vi "cRIO IV PID test.vi"(1 "AI Chan":i32, 2 "AO Channel":string(combo)="AO0", 7 "Voltage target V":dbl=1e-05, 12 "delay s":dbl=0.05 format="%.3f", 13 "error":dbl) -> (4 "I Output uA":dbl, 15 "error out":errorcluster)   [LabVIEW 2021]
uses:
  <vilib>/addons/control/pid/NI_PID_pid.lvlib
  <vilib>/addons/control/pid/pid.llb/PID (DBL).vi
panel:
  in  "Init Current uA":dbl=3.0 format="%#_13g"
  out "Voltage":cluster{"t0":dbl, "dt":dbl, dbl[][]}(graph)={"t0"=0.0, "dt"=0.23150301830064327, [[-6.2742919921875e-06, 7.0286865234375e-06, 7.5959472656250004e-06, 7.587646484375001e-06, 6.8331298828125e-06, 8.3389892578125e-06, 7.4207763671875e-06, 8.2294921875e-06, 6.97802734375e-06, 8.307373046875e-06, 7.221801757812501e-06, 7.378784179687501e-06, 8.218017578125e-06, 7.3470458984375005e-06, 8.3358154296875e-06, 7.828613281250001e-06, 9.2227783203125e-06, 9.056640625e-06, 8.68896484375e-06, 7.5644531249999994e-06, 8.111450195312501e-06, 9.3924560546875e-06, 9.149658203125e-06, 8.9468994140625e-06, 8.8182373046875e-06, 9.553344726562501e-06, 7.7969970703125e-06, 7.2528076171875e-06, 8.03564453125e-06, 9.9212646484375e-06, 9.2659912109375e-06, 8.3221435546875e-06, 8.722412109375e-06, 7.700927734375e-06, 9.4189453125e-06, 7.7850341796875e-06, 7.683349609375e-06, 1.14346923828125e-05, 1.01173095703125e-05, 9.098388671875e-06, 8.264038085937501e-06, 1.0583740234375e-05, 9.461791992187501e-06, 9.5201416015625e-06, 7.613403320312501e-06, 8.979125976562501e-06, 1.012158203125e-05, 8.5411376953125e-06, 8.268920898437501e-06, 8.615234375e-06, 8.764404296875e-06, 9.4747314453125e-06, 8.604370117187501e-06, 7.9896240234375e-06, 8.267822265625e-06, 8.7490234375e-06, 8.952026367187501e-06, 9.116943359375e-06, 1.1099365234375e-05, 9.396484375e-06, 9.9132080078125e-06, 1.0455322265625e-05, 1.02037353515625e-05, 9.993408203125e-06, 9.0792236328125e-06, 1.05933837890625e-05, 8.10009765625e-06, 1.131103515625e-05, 9.5404052734375e-06, 8.3836669921875e-06, 9.6424560546875e-06, 8.5926513671875e-06, 1.0763916015625e-05, 1.0721557617187499e-05, 9.448974609375e-06, 1.0819946289062501e-05, 8.394897460937502e-06, 1.03946533203125e-05, 9.9185791015625e-06, 9.932739257812501e-06, 9.6884765625e-06, 9.885986328125e-06, 9.747802734375e-06, 9.4522705078125e-06, 9.875122070312501e-06, 1.064501953125e-05, 1.02010498046875e-05, 9.4254150390625e-06, 1.05379638671875e-05, 1.062939453125e-05, 1.03377685546875e-05, 7.7686767578125e-06, 1.03857421875e-05, 8.9049072265625e-06, 1.01602783203125e-05, 1.0444458007812501e-05, 9.0526123046875e-06, 9.9517822265625e-06, 9.619873046875e-06, 9.9910888671875e-06, 9.627685546875001e-06, 1.16241455078125e-05, 1.01810302734375e-05, 8.827880859375e-06, 9.647827148437501e-06, 8.648193359375e-06, 9.631225585937501e-06, 1.1260375976562501e-05, 9.3602294921875e-06, 1.1323364257812501e-05, 1.00931396484375e-05, 9.7305908203125e-06, 1.0537109375000001e-05, 9.133178710937501e-06, 1.06405029296875e-05, 9.4534912109375e-06, 9.677490234375e-06, 1.0020385742187501e-05, 1.0294677734375e-05, 9.501953125e-06, 1.1838745117187502e-05, 1.01229248046875e-05, 1.0786132812500001e-05, 9.9029541015625e-06, 9.881469726562501e-06, 1.03533935546875e-05, 1.02386474609375e-05, 9.5933837890625e-06, 1.1360473632812501e-05, 8.740966796875e-06, 9.8046875e-06, 9.3798828125e-06, 9.642578124999999e-06, 1.087841796875e-05, 9.199951171875e-06, 1.0077880859375e-05, 1.04891357421875e-05, 9.737548828125001e-06, 9.2452392578125e-06, 9.141235351562501e-06, 1.0398071289062499e-05, 8.7894287109375e-06, 9.27197265625e-06, 9.757934570312501e-06, 1.03651123046875e-05, 9.6182861328125e-06, 9.383544921875001e-06, 1.01751708984375e-05, 1.06143798828125e-05, 8.880126953125e-06, 9.0814208984375e-06, 9.64013671875e-06, 9.750732421875e-06, 1.0253662109375e-05, 1.0913940429687502e-05, 9.9195556640625e-06, 1.0969360351562501e-05, 1.1051513671875e-05, 1.05164794921875e-05, 1.0513549804687501e-05, 1.0940307617187501e-05, 9.00634765625e-06, 9.565185546875001e-06, 1.08887939453125e-05, 9.060424804687501e-06, 1.09468994140625e-05, 9.7672119140625e-06, 9.77978515625e-06, 9.439208984375e-06, 8.5277099609375e-06, 1.17899169921875e-05, 1.0476074218750001e-05, 9.598754882812501e-06, 9.685546875000001e-06, 9.630859375000001e-06, 8.735229492187501e-06, 1.0571533203125e-05, 1.01201171875e-05, 9.3568115234375e-06, 1.1734130859375e-05, 1.00394287109375e-05, 9.65185546875e-06, 1.0709838867187501e-05, 9.6763916015625e-06, 1.07955322265625e-05, 8.813720703125e-06, 1.09769287109375e-05, 9.6085205078125e-06, 1.07159423828125e-05, 9.62841796875e-06, 1.0301025390625e-05, 9.542236328125e-06, 1.00299072265625e-05, 9.475219726562501e-06, 1.0421630859375e-05, 1.03519287109375e-05, 9.370117187500001e-06, 9.962646484375e-06, 9.717651367187501e-06, 1.0513427734375001e-05, 9.867187500000002e-06, 1.02030029296875e-05, 9.1756591796875e-06, 1.0221191406250002e-05, 8.7371826171875e-06, 9.9151611328125e-06, 9.8636474609375e-06, 1.0983642578125e-05, 1.06876220703125e-05, 9.659912109375001e-06, 8.753662109375001e-06, 9.053833007812502e-06, 1.0186401367187501e-05, 1.0432128906250001e-05, 1.0882812500000001e-05, 1.1218994140625e-05, 1.1887451171875001e-05, 1.0174072265625e-05, 9.899658203125e-06, 1.0531494140625e-05, 9.444824218750001e-06, 8.6407470703125e-06, 9.7640380859375e-06, 9.9656982421875e-06, 1.0595336914062502e-05, 9.55712890625e-06, 1.1597534179687501e-05, 9.322753906250001e-06, 1.0935424804687501e-05, 9.472045898437501e-06, 1.0580322265625e-05, 1.0116943359375001e-05, 9.96728515625e-06, 1.1901245117187501e-05, 1.0048583984375e-05, 1.0146484375000002e-05, 1.0034179687500001e-05, 1.044482421875e-05, 9.5802001953125e-06, 1.0305175781250001e-05, 9.824462890625001e-06, 9.204833984375e-06, 9.7882080078125e-06, 8.905517578125e-06, 8.972412109375e-06, 1.04232177734375e-05, 1.0131591796875e-05, 1.0323852539062501e-05, 1.0559326171875e-05, 1.06358642578125e-05, 1.0219482421875e-05, 1.0810424804687502e-05, 9.529907226562502e-06, 1.01871337890625e-05, 9.165283203125001e-06, 9.7891845703125e-06, 1.0254150390625001e-05, 1.0550781250000001e-05, 1.0967407226562501e-05, 9.429077148437499e-06, 9.159179687500002e-06, 9.6815185546875e-06, 1.1452514648437502e-05, 1.0664794921875e-05, 9.7794189453125e-06, 9.3082275390625e-06, 1.2046142578125e-05, 9.310546875e-06, 1.092138671875e-05, 9.867431640625e-06, 9.5145263671875e-06, 1.0375e-05, 1.0604858398437501e-05, 9.5135498046875e-06, 1.0877685546875001e-05, 8.9964599609375e-06, 9.785400390625001e-06, 1.0837646484375002e-05, 9.8760986328125e-06, 9.861572265625001e-06, 1.04326171875e-05, 1.1680419921875001e-05, 9.5611572265625e-06, 8.8084716796875e-06, 1.0350341796875e-05, 1.10693359375e-05, 8.979736328125e-06, 1.01485595703125e-05, 1.1346923828125e-05, 8.6527099609375e-06, 9.1024169921875e-06, 8.1697998046875e-06, 1.1321289062500001e-05, 8.2783203125e-06, 9.943603515625e-06, 8.751220703125e-06, 1.04207763671875e-05, 1.1733642578125002e-05, 1.1821533203125e-05, 1.08138427734375e-05, 1.00948486328125e-05, 9.882446289062502e-06, 9.6370849609375e-06, 8.97802734375e-06, 9.022216796875e-06, 9.816650390625e-06], [1e-05, 1e-05, 1e-05, 1e-05, 1e-05, 1e-05, 1e-05, 1e-05, 1e-05, 1e-05, 1e-05, 1e-05, 1e-05, 1e-05, 1e-05, 1e-05, 1e-05, 1e-05, 1e-05, 1e-05, 1e-05, 1e-05, 1e-05, 1e-05, 1e-05, 1e-05, 1e-05, 1e-05, 1e-05, 1e-05, 1e-05, 1e-05, 1e-05, 1e-05, 1e-05, 1e-05, 1e-05, 1e-05, 1e-05, 1e-05, 1e-05, 1e-05, 1e-05, 1e-05, 1e-05, 1e-05, 1e-05, 1e-05, 1e-05, 1e-05, 1e-05, 1e-05, 1e-05, 1e-05, 1e-05, 1e-05, 1e-05, 1e-05, 1e-05, 1e-05, 1e-05, 1e-05, 1e-05, 1e-05, 1e-05, 1e-05, 1e-05, 1e-05, 1e-05, 1e-05, 1e-05, 1e-05, 1e-05, 1e-05, 1e-05, 1e-05, 1e-05, 1e-05, 1e-05, 1e-05, 1e-05, 1e-05, 1e-05, 1e-05, 1e-05, 1e-05, 1e-05, 1e-05, 1e-05, 1e-05, 1e-05, 1e-05, 1e-05, 1e-05, 1e-05, 1e-05, 1e-05, 1e-05, 1e-05, 1e-05, 1e-05, 1e-05, 1e-05, 1e-05, 1e-05, 1e-05, 1e-05, 1e-05, 1e-05, 1e-05, 1e-05, 1e-05, 1e-05, 1e-05, 1e-05, 1e-05, 1e-05, 1e-05, 1e-05, 1e-05, 1e-05, 1e-05, 1e-05, 1e-05, 1e-05, 1e-05, 1e-05, 1e-05, 1e-05, 1e-05, 1e-05, 1e-05, 1e-05, 1e-05, 1e-05, 1e-05, 1e-05, 1e-05, 1e-05, 1e-05, 1e-05, 1e-05, 1e-05, 1e-05, 1e-05, 1e-05, 1e-05, 1e-05, 1e-05, 1e-05, 1e-05, 1e-05, 1e-05, 1e-05, 1e-05, 1e-05, 1e-05, 1e-05, 1e-05, 1e-05, 1e-05, 1e-05, 1e-05, 1e-05, 1e-05, 1e-05, 1e-05, 1e-05, 1e-05, 1e-05, 1e-05, 1e-05, 1e-05, 1e-05, 1e-05, 1e-05, 1e-05, 1e-05, 1e-05, 1e-05, 1e-05, 1e-05, 1e-05, 1e-05, 1e-05, 1e-05, 1e-05, 1e-05, 1e-05, 1e-05, 1e-05, 1e-05, 1e-05, 1e-05, 1e-05, 1e-05, 1e-05, 1e-05, 1e-05, 1e-05, 1e-05, 1e-05, 1e-05, 1e-05, 1e-05, 1e-05, 1e-05, 1e-05, 1e-05, 1e-05, 1e-05, 1e-05, 1e-05, 1e-05, 1e-05, 1e-05, 1e-05, 1e-05, 1e-05, 1e-05, 1e-05, 1e-05, 1e-05, 1e-05, 1e-05, 1e-05, 1e-05, 1e-05, 1e-05, 1e-05, 1e-05, 1e-05, 1e-05, 1e-05, 1e-05, 1e-05, 1e-05, 1e-05, 1e-05, 1e-05, 1e-05, 1e-05, 1e-05, 1e-05, 1e-05, 1e-05, 1e-05, 1e-05, 1e-05, 1e-05, 1e-05, 1e-05, 1e-05, 1e-05, 1e-05, 1e-05, 1e-05, 1e-05, 1e-05, 1e-05, 1e-05, 1e-05, 1e-05, 1e-05, 1e-05, 1e-05, 1e-05, 1e-05, 1e-05, 1e-05, 1e-05, 1e-05, 1e-05, 1e-05, 1e-05, 1e-05, 1e-05, 1e-05, 1e-05, 1e-05, 1e-05, 1e-05, 1e-05, 1e-05, 1e-05, 1e-05, 1e-05, 1e-05, 1e-05, 1e-05, 1e-05, 1e-05, 1e-05, 1e-05, 1e-05, 1e-05, 1e-05, 1e-05, 1e-05, 1e-05, 1e-05, 1e-05, 1e-05, 1e-05, 1e-05, 1e-05]]}
  out "Current":T1(graph)={"t0"=0.0, "dt"=0.23150301830064327, "Current array"=[3.006509716796875, 3.0076982428290204, 3.008659864605964, 3.00962480673273, 3.0108915555432136, 3.011555960640877, 3.012587650927396, 3.0132958549192814, 3.0145046448855526, 3.015181696606828, 3.0162929768781503, 3.017341464222326, 3.0180542582410417, 3.019115440965791, 3.019781115911303, 3.0206496717457356, 3.020960561587261, 3.021337906520166, 3.021862321782928, 3.0228365417620404, 3.0235919629463752, 3.0238349818062042, 3.024175119817897, 3.024596361359919, 3.025069067762951, 3.0252477312098036, 3.02612893373961, 3.0272278120888694, 3.028013555708861, 3.0280450512977475, 3.028338656267904, 3.029009800319169, 3.029520836971361, 3.030440467401184, 3.0306728908220024, 3.0315588787175365, 3.032485540476193, 3.0319116651322875, 3.031864742901392, 3.032225389035931, 3.0329197754252206, 3.032686280964038, 3.032901565799378, 3.033093510798843, 3.03404815113298, 3.0344565024309724, 3.034407871314046, 3.0349914179418387, 3.0356838513130504, 3.036237759317731, 3.036731999373934, 3.0369421085843813, 3.037500362340937, 3.038304514561335, 3.0389973875138043, 3.0394977800205947, 3.039916971373285, 3.0402701959440295, 3.039830451763102, 3.040071859922092, 3.0401065786332917, 3.0399244516385187, 3.0398429594042793, 3.039845598027892, 3.0402139104867927, 3.039976558885723, 3.04073652174787, 3.0402121096145653, 3.040395949427809, 3.041042484569587, 3.041185504101611, 3.041748445522266, 3.041442881088515, 3.041154260002669, 3.041374672118631, 3.041046695560642, 3.041688738539966, 3.0415308791848856, 3.041563449514887, 3.041590355783536, 3.041714967133234, 3.041760574579968, 3.0418614554670294, 3.0420805492508913, 3.042130502414945, 3.0418724965906057, 3.0417920786503556, 3.0420219146192404, 3.041806731057158, 3.0415549752204347, 3.041419869766867, 3.0423124010466727, 3.0421581061688574, 3.0425961452808954, 3.042532035962653, 3.0423542547647404, 3.0427332118519614, 3.0427525009781196, 3.0429045537794606, 3.042908120255681, 3.0430570480629706, 3.042407391876219, 3.0423349817692773, 3.0428038314356147, 3.0429447025980987, 3.0434854272893648, 3.043632939103291, 3.0431287907540807, 3.043384700993828, 3.042855357322046, 3.042818103483074, 3.042925869176714, 3.042711027446411, 3.0430577579842795, 3.0428015588363957, 3.043020164375286, 3.043149170311513, 3.043141018046948, 3.0430231489830746, 3.0432223697645218, 3.042486873738742, 3.042437705822814, 3.0421232546967416, 3.042162075049723, 3.042209489154369, 3.0420681337259516, 3.0419726767304627, 3.0421353252050207, 3.0415911377347116, 3.0420947529979934, 3.042172879991262, 3.0424209288658304, 3.0425638996229516, 3.0422125344385478, 3.0425325559722887, 3.0425014056366084, 3.042305753343423, 3.0424107358141113, 3.0427126421207817, 3.043056150002415, 3.0428969235126067, 3.043381154060324, 3.04367236704489, 3.043769195271324, 3.043623152403058, 3.04377584000367, 3.044022424096366, 3.0439523578018455, 3.0437066079074775, 3.0441545591888883, 3.044521992907921, 3.0446659403087035, 3.044765649432941, 3.044664186682145, 3.0442986125942055, 3.044330792406079, 3.043943050336085, 3.043522446922355, 3.0433158571683876, 3.0431104392814636, 3.0427343182583098, 3.043131781219943, 3.04330570903636, 3.0429501934898946, 3.0433260256000714, 3.0429472678664418, 3.0430403851272954, 3.0431284730947734, 3.043352791537035, 3.0439417096043764, 3.0432257448567643, 3.0430353172010234, 3.0431958172790794, 3.043321600565789, 3.0434692588577787, 3.043975169115514, 3.043746557894229, 3.043698513073852, 3.0439557905231394, 3.0432621402296256, 3.0432463707817887, 3.043385630633211, 3.0431016971224643, 3.043231142514984, 3.0429129316538583, 3.043387445405126, 3.042996675954886, 3.0431532697813735, 3.0428668948553548, 3.043015529692301, 3.0428951215610427, 3.0430782290559946, 3.043066268194876, 3.0432761823375802, 3.043107532027956, 3.042966762571732, 3.04321871772703, 3.043233661168731, 3.043346602659777, 3.043141233602163, 3.0431943606353595, 3.043113161496139, 3.043442899861717, 3.043354425341327, 3.0438595543446056, 3.043893491952041, 3.0439480350299344, 3.04355458005441, 3.043279533269107, 3.0434155704654953, 3.043914107674133, 3.044292576540325, 3.0442180180686322, 3.0440451685765395, 3.043692045636795, 3.0432044500245703, 3.0424494715758597, 3.042379844673732, 3.0424199833960346, 3.042207387740009, 3.042429460052916, 3.0429731632399806, 3.043067550033112, 3.0430812727658303, 3.0428431400254667, 3.043020290487051, 3.0423812788303457, 3.04265217927591, 3.0422780113601062, 3.0424891950036566, 3.0422570680999272, 3.0422102927533152, 3.042223380687303, 3.041462884622491, 3.041443452995752, 3.0413848612112573, 3.0413711913003674, 3.0411932635732795, 3.0413611854553735, 3.041239117103977, 3.0413093339078303, 3.041627402281677, 3.041712121053922, 3.0421499160081256, 3.0425609531662103, 3.042391668063335, 3.0423390333468023, 3.042209494329879, 3.041985765853014, 3.0417314221325484, 3.041643631139856, 3.0413194631860896, 3.0415075022609463, 3.041432650712987, 3.0417665394044007, 3.0418508675570086, 3.041749209381157, 3.041528898855343, 3.041141937927185, 3.041370309027216, 3.0417066391225194, 3.041834033679897, 3.0412530297910196, 3.0409871137764224, 3.0410753481490214, 3.041352059091163, 3.040533604007225, 3.0408093871940642, 3.040440834441613, 3.040493863714323, 3.0406880551011786, 3.0405380570357616, 3.040296115603407, 3.0404906976076385, 3.0401396253119755, 3.0405410432516584, 3.0406268850288685, 3.04029182836377, 3.0403413908337873, 3.0403967638527045, 3.040223718900601, 3.0395515528384407, 3.039727091844824, 3.040203705082539, 3.040063570279871, 3.039635837809997, 3.0400439451834944, 3.0399845232668437, 3.0394457556355263, 3.039984673551087, 3.0403437086714717, 3.041075790687906, 3.040547277005143, 3.04123595082547, 3.041258511378268, 3.0417580250661387, 3.041589716494774, 3.0408962614224078, 3.0401676500726067, 3.039842114874344, 3.039804177325319, 3.0398512007139695, 3.0399963686375773, 3.040405159618747, 3.0407962748340984, 3.04086961662091]}
  in  "Average":i32=200
  out "Current uA":dbl=3.04086961662091
  in  "Stop":bool
  in  "I Scale factor":dbl=10.0
  in  "V Scale factor":dbl=0.0001
  in  "PID gains":T2={"proportional gain (Kc)"=400.0, "integral time (Ti, min)"=100000.0, "derivative time (Td, min)"=0.0} {"derivative time (Td, min)" format="%.3f"; "integral time (Ti, min)" format="%.3f"; "proportional gain (Kc)" format="%.3f"}
  # "Voltage x factor=actual"
  # "Voltage x factor=uA"
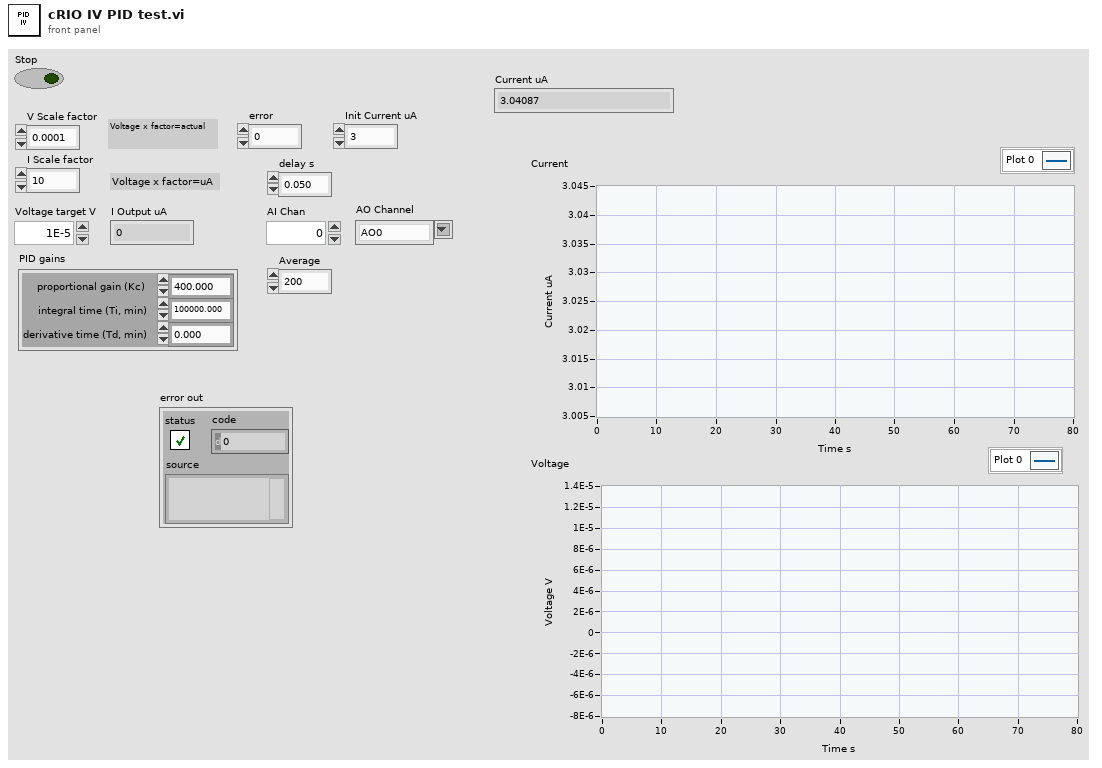
[diagram p1: front panel]
types:
  T1 = cluster{"t0":dbl, "dt":dbl, "Current array":dbl[]}
  T2 = cluster{"proportional gain (Kc)":dbl, "integral time (Ti, min)":dbl, "derivative time (Td, min)":dbl}
  T3 = cluster{"AI0":dbl, "AI1":dbl, "AI2":dbl, "AI3":dbl}
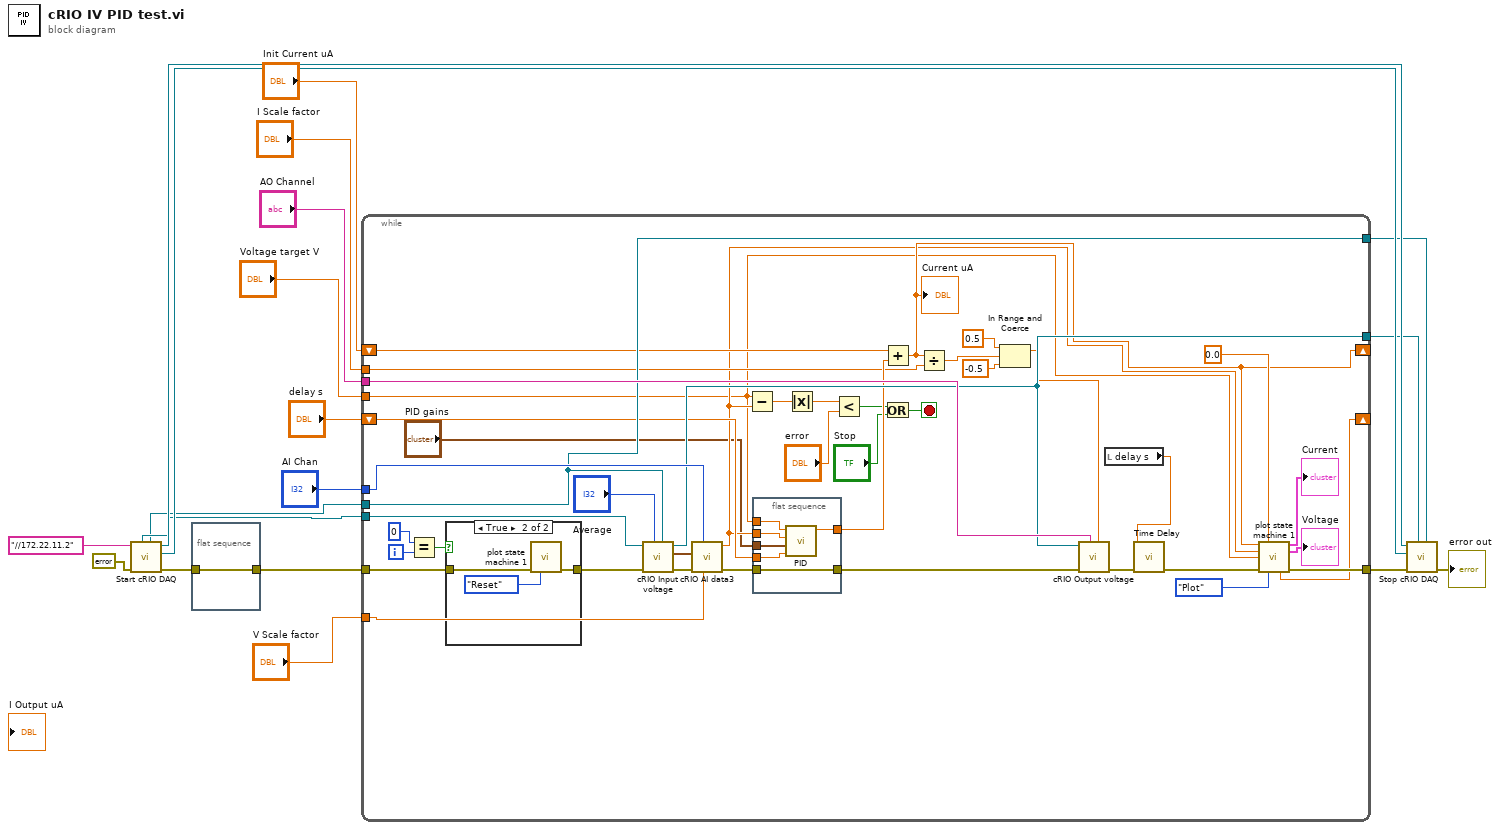
[diagram p0: block diagram]
diagram:
  n1 = call "Start cRIO DAQ.vi"("error in (no error)"=errorcluster {"status"=FALSE, "code"=0, "source"=""}, "cRIO IP"="//172.22.11.2") -> ("error out"=w3:errorcluster, "vi reference"=w9:refnum<vi>, "application reference"=w10:refnum<vi>, "DAQ_AI_Reader endpoint"=w7:refnum<k21>, "DAQ_CMD_Writer endpoint"=w8:refnum<k21>)  [unwired: 5 in]
  n2 = flat-sequence {
    tunnel: [w20] -> w2
    tunnel: w3 -> [w20]
    frame #0 {
    }
  }
  n3 = while {
    tunnel: w2 -> [w33]
    tunnel: [w37] -> w12
    tunnel: "Voltage target V" -> [w26]
    tunnel: w8 -> [w59]
    tunnel: w7 -> [w50]
    tunnel: "V Scale factor" -> [w61]
    tunnel: "AI Chan" -> [w58]
    tunnel: "AO Channel" -> [w57]
    tunnel: "I Scale factor" -> [w48]
    tunnel: [w51] -> w5
    tunnel: [w50] -> w4
    shift-right: [w28] -> _
    shift-left: "Init Current uA" -> [w39]
    shift-right: [w22] -> _
    shift-left: "delay s" -> [w29]
    i -> [w36]
    stop <- w41 stop-if-true
    n4 = Equal?(x=0, y=w36) -> (x = y?=w34:bool)
    n5 = case shown="True" w34 {
      tunnel: w33 -> [w64 w67]
      tunnel: [w64 w66] -> w32
      frame False {
      }
      frame True {
        n6 = call "plot state machine 1.vi"("error in"=w67, "Enum"=enum16{"Reset", "Plot"}."Reset") -> ("error out"=w66:errorcluster)  [unwired: 10 in, 3 out]
      }
    }
    n7 = call "cRIO Input voltage.vi"("DAQ_AI_Reader endpoint"=w50, "Average"="Average", "error in (no error)"=w32, "DAQ_CMD_Writer endpoint"=w59) -> ("error out"=w62:errorcluster, "output cluster"=w63:T3, "DAQ_CMD_Writer endpoint out"=w51:refnum<k21>)  [unwired: 5 in]
    n8 = call "cRIO AI data3.vi"("Scale factor"=w61, "Chan"=w58, "error in (no error)"=w62, "Input cluster"=w63) -> ("error out"=w60:errorcluster, "Output"=w27:dbl)  [unwired: 6 in]
    n9 = Subtract(x=w26, y=w27) -> (x-y=w54:dbl)
    n10 = flat-sequence {
      tunnel: "PID gains" -> [w73]
      tunnel: w29 -> [w72]
      tunnel: w26 -> [w68]
      tunnel: w27 -> [w71]
      tunnel: w60 -> [w70]
      tunnel: [w70] -> w56
      tunnel: [w69] -> w49
      frame #0 {
        n11 = call-poly <vilib>:"PID.vi"("dt (s)"=w72, "PID gains"=w73, "process variable"=w71, "setpoint"=w68) -> ("output"=w69:dbl)  [unwired: 6 in, 1 out]
      }
    }
    n12 = Absolute Value(x=w54) -> (abs(x)=w53:dbl)
    n13 = Less?(x=w53, y="error") -> (x < y?=w43:bool)
    n14 = Add(x=w39, y=w49) -> (x+y=w28:dbl)
    "Current uA" <- w28
    n15 = Or(x=w43, y="Stop") -> (x .or. y?=w41:bool)
    n16 = Divide(x=w28, y=w48) -> (x/y=w47:dbl)
    n17 = In Range and Coerce(upper limit=0.5, x=w47, lower limit=-0.5) -> (coerced(x)=w46:dbl)  [unwired: 1 out]
    n18 = call "cRIO Output voltage.vi"("Voltage"=w46, "AO Channel"=w57, "error in (no error)"=w56, "DAQ_CMD_Writer endpoint"=w51) -> ("error out"=w55:errorcluster)  [unwired: 6 in, 1 out]
    n19 = local read "delay s"() -> (w21:dbl)
    n20 = call "Time Delay"("error in (no error)"=w55, "Delay Time (s)"=w21) -> ("error out"=w38:errorcluster)  [unwired: 9 in]
    n21 = call "plot state machine 1.vi"("current"=w28, "t0"=0.0, "Voltage"=w27, "Voltage target"=w26, "error in"=w38, "Enum"=enum16{"Reset", "Plot"}."Plot") -> ("Current plot"=→"Current":T1, "Voltage plot"=→"Voltage":cluster{"t0":dbl, "dt":dbl, dbl[][]}, "dt"=w22:dbl, "error out"=w37:errorcluster)  [unwired: 6 in]
  }
  n22 = call "Stop cRIO DAQ.vi"("DAQ_AI_Reader endpoint"=w4, "DAQ_CMD_Writer endpoint"=w5, "error in (no error)"=w12, "VI reference"=w9, "application reference"=w10) -> ("error out"=→"error out":errorcluster)  [unwired: 6 in]
